vi "GetVisible.vi"(8 "Error In":errorcluster, 11 "reference in":refnum<class "Clippy.lvclass">) -> (0 "Error Out":errorcluster, 2 "Visible":bool, 3 "reference out":refnum<class "Clippy.lvclass">)   [LabVIEW 2020, in "Clippy.lvclass"]
uses:
  Clippy.lvclass
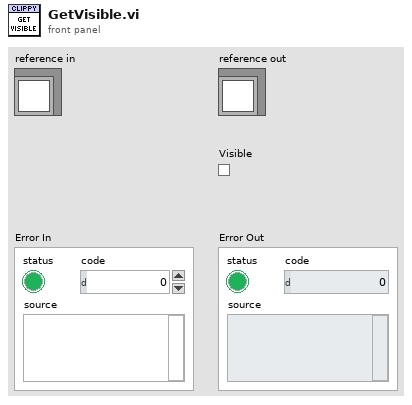
[diagram p1: front panel]
types:
  T1 = typedef "Clippy.lvclass/ObjectAttributes.ctl" = cluster{"ClippyPictureRef":refnum<vi>, "LastAnimation":T2, "LastAnimated":timestamp, "Visible":bool, "AnswerRef":refnum<vi>}
  T2 = typedef "Clippy.lvclass/AnimationTypes.ctl" = enum16{"Congratulate", "LookRight", "SendMail", "Thinking", "Explain", "IdleRopePile", "IdleAtom", "Print", "Hide", "GetAttention", "Save", "GetTechy", "GestureUp", "Idle1_1", "Processing", "Alert", "LookUpRight", "IdleSideToSide", "GoodBye", "LookLeft", "IdleHeadScratch", "LookUpLeft", "CheckingSomething", "Hearing_1", "GetWizardy", "IdleFingerTap", "GestureLeft", "Wave", "GestureRight", "Writing", "IdleSnooze", "LookDownRight", "GetArtsy", "Show", "LookDown", "Searching", "EmptyTrash", "Greeting", "LookUp", "GestureDown", "RestPose", "IdleEyeBrowRaise", "LookDownLeft"}
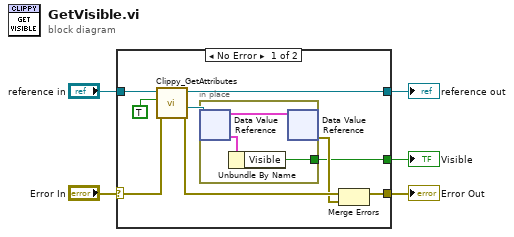
[diagram p0: block diagram]
diagram:
  n1 = case shown="No Error" "Error In" {
    selector: "Error In" -> [w14 w18]
    tunnel: [w12 w18] -> w4
    tunnel: [w9 w17] -> w2
    tunnel: "reference in" -> [w10 w17]
    tunnel: [w6 _] -> w1
    frame No Error {
      n2 = call "Clippy_GetAttributes.vi"("error in (no error)"=w14, "OnlyGetDvrReference(False)"=TRUE, "reference in"=w10) -> ("error out"=w13:errorcluster, "DataRef"=w7:refnum<data-value>, "reference out"=w9:refnum<class "Clippy.lvclass">)  [unwired: 5 in, 1 out]
      n3 = in-place {
        in-place-border: [w16] -> w6
        n4 = in-place-dvr #1(w7) -> (w15:T1)  [unwired: 1 out]
        n5 = Unbundle By Name(w15) -> ("Visible"=w16:bool)
        n6 = in-place-dvr #1(w15) -> (w11:errorcluster)  [unwired: 1 out]
      }
      n7 = Merge Errors(w13, w11) -> (w12:errorcluster)
    }
    frame Error {
    }
  }
  "Error Out" <- w4
  "reference out" <- w2
  "Visible" <- w1
